vi "CopyInstruction.vi"() -> (1 "Instruction to copy":T2={"Duration"=0.01, "Comment"="", "Steps"=1, "Edit Potential"=FALSE, "Output Bits"=[], "Macro Path"=path "", "Potentials"=[], "Inherit?"=FALSE} {"Steps" min=1 max=100000 step=1; "Duration" min=0.001 step=0.001 format="%_6p"}, 2 "Insert Index":u32=3)   [LabVIEW 2018]
uses:
  Executor Files/RT/Instruction.ctl
  Instructions.ctl
panel:
  in  "Done":bool
  in  "Destination index":u32=3
  in  "Source index":u32=3
  in  "Open Path":path=path "C:/CuspControl/Macros/Test/5-10-15-etc.mac"
  in  "Instructions":T1=[{"Duration"=0.001, "Comment"="", "Steps"=1, "Edit Potential"=FALSE, "Output Bits"=[FALSE, FALSE, FALSE, FALSE, FALSE, FALSE, FALSE, FALSE, FALSE, FALSE, FALSE, FALSE, FALSE, FALSE, FALSE, FALSE, FALSE, FALSE, FALSE, FALSE, FALSE, FALSE, FALSE, FALSE, FALSE, FALSE, FALSE, FALSE, FALSE, FALSE, FALSE, FALSE, FALSE, FALSE, FALSE, FALSE, FALSE, FALSE], "Macro Path"=path "", "Potentials"=[0.0, 0.0, 0.0, 0.0, 0.0, 0.0, 0.0, 0.0, 0.0, 0.0, 0.0, 0.0, 0.0, 0.0, 0.0, 0.0, 0.0, 0.0, 0.0, 0.0, 0.0, 0.0], "Inherit?"=FALSE}, {"Duration"=0.01, "Comment"="", "Steps"=100, "Edit Potential"=FALSE, "Output Bits"=[FALSE, FALSE, FALSE, FALSE, FALSE, FALSE, FALSE, FALSE, FALSE, FALSE, FALSE, FALSE, FALSE, FALSE, FALSE, FALSE, FALSE, FALSE, FALSE, FALSE, FALSE, FALSE, FALSE, FALSE, FALSE, FALSE, FALSE, FALSE, FALSE, FALSE, FALSE, FALSE, FALSE, FALSE, FALSE, FALSE, FALSE, FALSE], "Macro Path"=path "", "Potentials"=[10.0, 10.0, 10.0, 10.0, 10.0, 10.0, 10.0, 10.0, 10.0, 0.0, 0.0, 0.0, 0.0, 0.0, 0.0, 0.0, 0.0, 0.0, 0.0, 0.0, 0.0, 0.0], "Inherit?"=TRUE}, {"Duration"=0.01, "Comment"="", "Steps"=100, "Edit Potential"=FALSE, "Output Bits"=[FALSE, FALSE, FALSE, FALSE, FALSE, FALSE, FALSE, FALSE, FALSE, FALSE, FALSE, FALSE, FALSE, FALSE, FALSE, FALSE, FALSE, FALSE, FALSE, FALSE, FALSE, FALSE, FALSE, FALSE, FALSE, FALSE, FALSE, FALSE, FALSE, FALSE, FALSE, FALSE, FALSE, FALSE, FALSE, FALSE, FALSE, FALSE], "Macro Path"=path "", "Potentials"=[0.0, 0.0, 0.0, 0.0, 0.0, 0.0, 0.0, 0.0, 0.0, 0.0, 0.0, 0.0, 0.0, 0.0, 0.0, 0.0, 0.0, 0.0, 0.0, 0.0, 0.0, 0.0], "Inherit?"=TRUE}, {"Duration"=0.01, "Comment"="", "Steps"=100, "Edit Potential"=FALSE, "Output Bits"=[FALSE, FALSE, FALSE, FALSE, FALSE, FALSE, FALSE, FALSE, FALSE, FALSE, FALSE, FALSE, FALSE, FALSE, FALSE, FALSE, FALSE, FALSE, FALSE, FALSE, FALSE, FALSE, FALSE, FALSE, FALSE, FALSE, FALSE, FALSE, FALSE, FALSE, FALSE, FALSE, FALSE, FALSE, FALSE, FALSE, FALSE, FALSE], "Macro Path"=path "", "Potentials"=[0.0, 0.0, 0.0, 0.0, 0.0, 0.0, 0.0, 0.0, 0.0, 0.0, 0.0, 0.0, 0.0, 0.0, 0.0, 0.0, 0.0, 0.0, 0.0, 0.0, 0.0, 0.0], "Inherit?"=TRUE}] {"Steps" min=1 max=100000 step=1; "Duration" min=0.001 step=0.001 format="%_6p"}
  # "0        2       4       6        8      10     12     14     16     18      20    22     24     26     28     30     32     34     36"
  # "0        2       4       6        8      10     12     14     16     18      20    22     24     26     28     30     32     34     36"
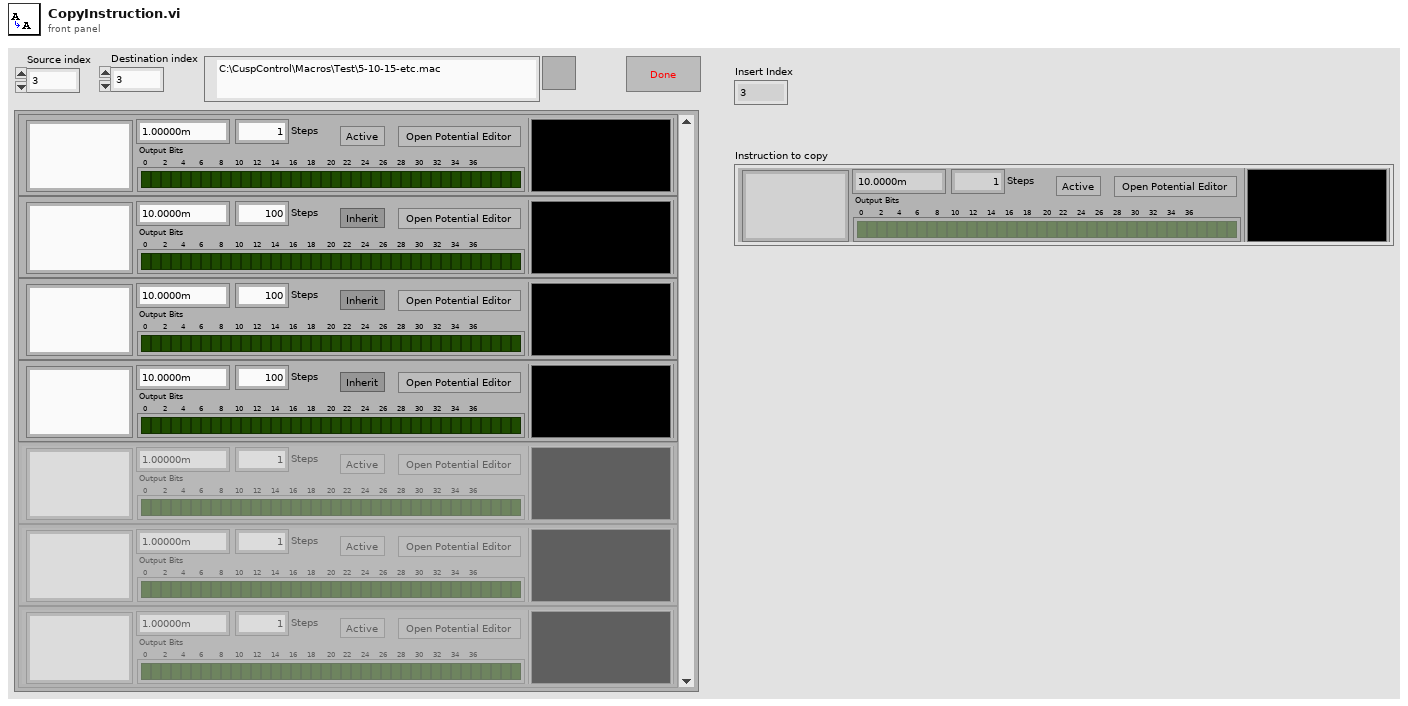
[diagram p1: front panel]
types:
  T1 = typedef "Instructions.ctl" = T2[]
  T2 = typedef "Instruction.ctl" = cluster{"Duration":dbl, "Comment":string, "Steps":i32, "Edit Potential":bool, "Output Bits":bool[], "Macro Path":path, "Potentials":dbl[], "Inherit?":bool}
  T3 = typedef "MacroSaveCluster.ctl" = cluster{"Instructions":T1, "Changes":bool[][], "Macro Description":string, "Total Time (s)":dbl, "Samples per sec":dbl}
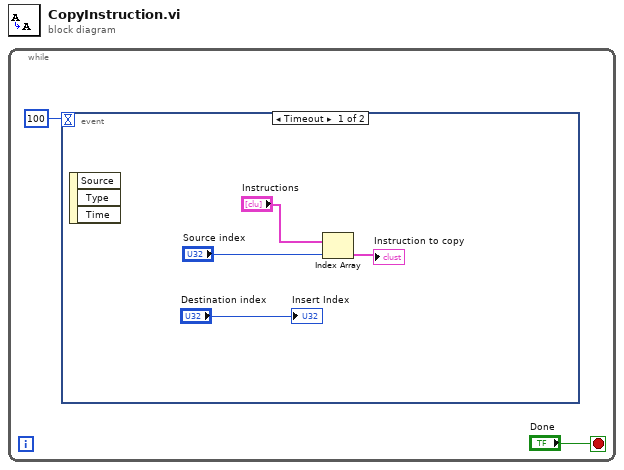
[diagram p0: block diagram]
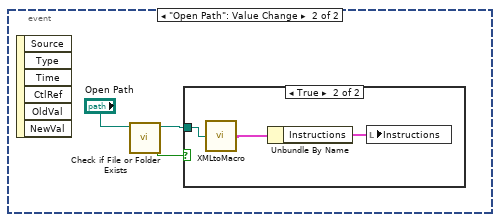
[diagram p2: hidden frame]
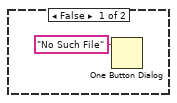
[diagram p3: hidden frame]
diagram:
  n1 = while {
    stop <- "Done" stop-if-true
    n2 = event shown="[0] Timeout" {
      selector: _ -> [_ _]
      dyn-events: _ -> [_ _]
      timeout: u32 100 ("milliseconds to wait") -> [_ _]
      event Timeout {
        n3 = event-data() -> ()  [unwired: 1 in, 3 out]
        n4 = Index Array(array="Instructions", index="Source index") -> (element=→"Instruction to copy":T2)
        "Insert Index" <- "Destination index"
      }
      event "Open Path": Value Change {
        n5 = event-data() -> ()  [unwired: 1 in, 6 out]
        n6 = call <vilib>:"Check if File or Folder Exists.vi"("path"="Open Path") -> ("file or folder exists?"=w7:bool, "dup path"=w8:path)  [unwired: 8 in, 1 out]
        n7 = case shown="True" w7 {
          tunnel: w8 -> [_ w11]
          frame False {
            n8 = One Button Dialog(message="No Such File") -> ()  [unwired: 1 in, 1 out]
          }
          frame True {
            n9 = call "XMLtoMacro.vi"("XML File Path"=w11) -> ("MacroSaveCluster"=w12:T3)
            n10 = Unbundle By Name(w12) -> ("Instructions"=w13:T1)
            n11 = local write "Instructions"(w13) -> ()
          }
        }
      }
    }
  }
